vi "SystemVolume.Devices.List.vi"(6 "Mode":i32(ring)=2 items=["Render", "Capture", "All"], 8 "error in (no error)":errorcluster, 11 "FriendlyName (\"\": All)":string) -> (0 "error out":errorcluster, 3 "Info":T1(array[cluster]))   [LabVIEW 2014]
uses:
  C:/Program Files (x86)/National Instruments/LabVIEW 2014/user.lib/dge-library/LabVIEW/System/SystemVolume/NAudio.dll
  NAudio.dll
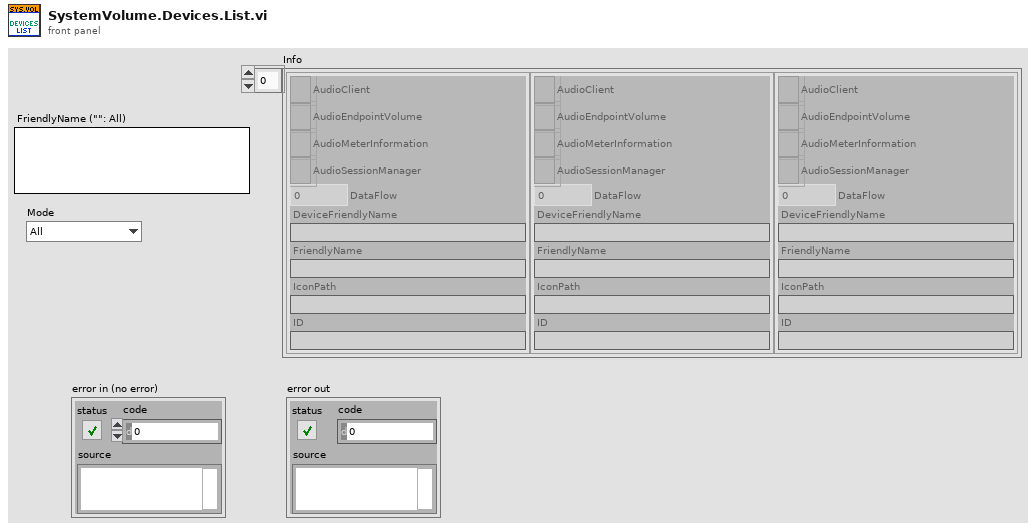
[diagram p1: front panel]
types:
  T1 = cluster{"AudioClient":refnum<k24>, "AudioEndpointVolume":refnum<k24>, "AudioMeterInformation":refnum<k24>, "AudioSessionManager":refnum<k24>, "DataFlow":i32, "DeviceFriendlyName":string, "FriendlyName":string, "IconPath":string, "ID":string}[]
  T2 = cluster{"AudioClient":refnum<k24>, "AudioEndpointVolume":refnum<k24>, "AudioMeterInformation":refnum<k24>, "AudioSessionManager":refnum<k24>, "DataFlow":i32, "DeviceFriendlyName":string, "FriendlyName":string, "IconPath":string, "ID":string}
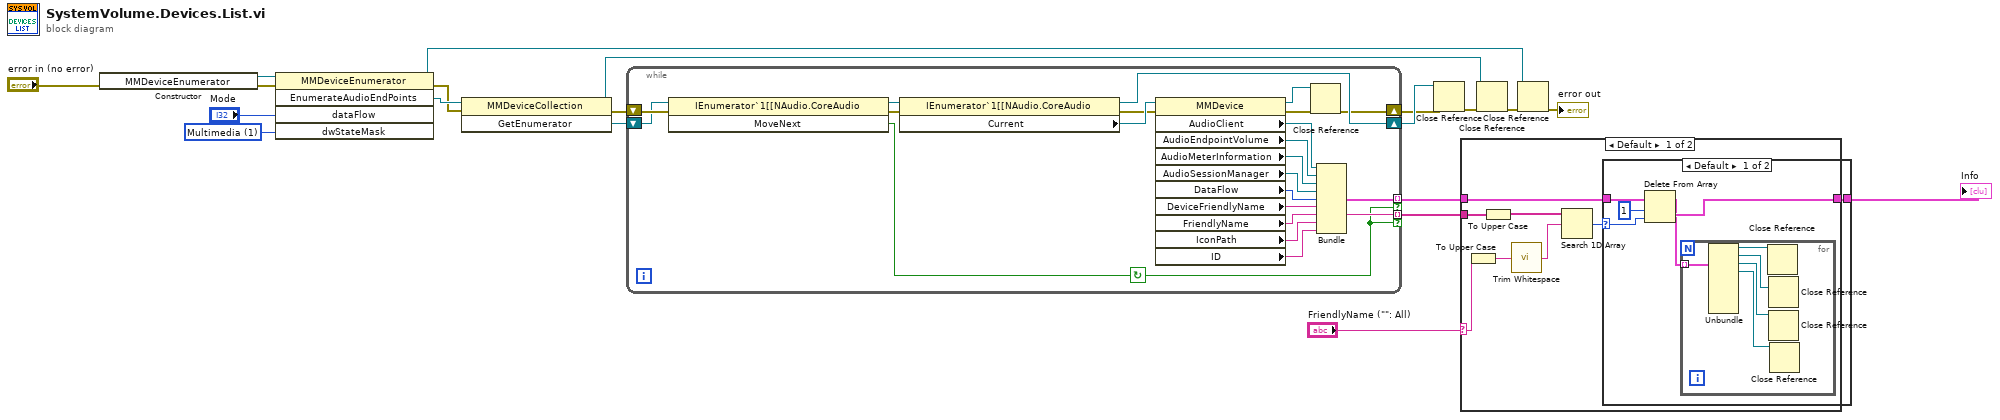
[diagram p0: block diagram]
diagram:
  w18 = 1 items=["Console", "Multimedia", "Communications"] ("role")
  n1 = constructor class="MMDeviceEnumerator"(error in="error in (no error)") -> (reference out=w20:refnum<k24>, error out=w17:errorcluster)  [unwired: 2 in, 1 out]
  n2 = invoke class="MMDeviceEnumerator" method="EnumerateAudioEndPoints"(reference=w20, error in=w17, "dataFlow"="Mode", "dwStateMask"=w18) -> (reference out=w6:refnum<k24>, error out=w13:errorcluster, "EnumerateAudioEndPoints"=w15:refnum<k24>)  [unwired: 1 in, 2 out]
  n3 = invoke class="MMDeviceCollection" method="GetEnumerator"(reference=w15, error in=w13) -> (reference out=w8:refnum<k24>, error out=w12:errorcluster, "GetEnumerator"=w14:refnum<k24>)  [unwired: 1 in]
  n4 = while {
    shift-right: [w33] -> w10
    shift-left: w12 -> [w39]
    shift-right: [w34] -> w11
    shift-left: w14 -> [w32]
    tunnel: [w23] -> w3 mode=indexing if=w21
    tunnel: [w22] -> w1 mode=indexing if=w21
    stop <- w21 continue-if-true
    n5 = invoke class="IEnumerator`1[[NAudio.CoreAudio" method="MoveNext"(reference=w32, error in=w39) -> (reference out=w40:refnum<k24>, error out=w38:errorcluster, "MoveNext"=w21:bool)  [unwired: 1 in]
    n6 = property class="IEnumerator`1[[NAudio.CoreAudio"(reference=w40, error in=w38) -> (reference out=w34:refnum<k24>, error out=w37:errorcluster, "Current"=w41:refnum<k24>)
    n7 = property class="MMDevice"(reference=w41, error in=w37) -> (reference out=w35:refnum<k24>, error out=w36:errorcluster, "AudioClient"=w31:refnum<k24>, "AudioEndpointVolume"=w30:refnum<k24>, "AudioMeterInformation"=w29:refnum<k24>, "AudioSessionManager"=w28:refnum<k24>, "DataFlow"=w27:i32, "DeviceFriendlyName"=w26:string, "FriendlyName"=w22:string, "IconPath"=w25:string, "ID"=w24:string)
    n8 = Close Reference(reference=w35, error in (no error)=w36) -> (error out=w33:errorcluster)
    n9 = Bundle("AudioClient"=w31, "AudioEndpointVolume"=w30, "AudioMeterInformation"=w29, "AudioSessionManager"=w28, "DataFlow"=w27, "DeviceFriendlyName"=w26, "FriendlyName"=w22, "IconPath"=w25, "ID"=w24) -> (w23:T2)  [unwired: 1 in]
  }
  n10 = Close Reference(reference=w11, error in (no error)=w10) -> (error out=w9:errorcluster)
  n11 = case shown="Default" "FriendlyName (\"\": All)" {
    selector: "FriendlyName (\"\": All)" -> [w49 _]
    tunnel: w3 -> [w43 w61]
    tunnel: [w42 w61] -> w2
    tunnel: w1 -> [w48 _]
    frame Default {
      n12 = To Upper Case(1:w49) -> (0:w47:string)
      n13 = To Upper Case(1:w48) -> (0:w46:string[])
      n14 = call <vilib>:"Trim Whitespace.vi"("string"=w47) -> ("trimmed string"=w45:string)  [unwired: 1 in]
      n15 = Search 1D Array(1D array=w46, element=w45) -> (index of element=w44:i32)  [unwired: 1 in]
      n16 = case shown="Default" w44 {
        selector: w44 -> [w54 _]
        tunnel: [w51 w60] -> w42
        tunnel: w43 -> [w53 w60]
        frame Default {
          n17 = Delete From Array(array=w53, length=1, index=w54) -> (deleted portion=w51:T1, array with subset deleted=w50:T1)
          n18 = for {
            tunnel: w50 -> [w59] mode=indexing
            n19 = Unbundle(w59) -> ("AudioClient"=w58:refnum<k24>, "AudioEndpointVolume"=w57:refnum<k24>, "AudioMeterInformation"=w56:refnum<k24>, "AudioSessionManager"=w55:refnum<k24>)  [unwired: 5 out]
            n20 = Close Reference(reference=w58) -> ()  [unwired: 1 in, 1 out]
            n21 = Close Reference(reference=w57) -> ()  [unwired: 1 in, 1 out]
            n22 = Close Reference(reference=w56) -> ()  [unwired: 1 in, 1 out]
            n23 = Close Reference(reference=w55) -> ()  [unwired: 1 in, 1 out]
          }
        }
        frame -1 {
        }
      }
    }
    frame "" {
    }
  }
  "Info" <- w2
  n24 = Close Reference(reference=w8, error in (no error)=w9) -> (error out=w7:errorcluster)
  n25 = Close Reference(reference=w6, error in (no error)=w7) -> (error out=→"error out":errorcluster)
